vi "BusyLock.vi"(7 "BusyLock":refnum<vi>, 9 "Timeout(250)":i32=250, 10 "ExitEvent":refnum<user-event>, 11 "Counter":refnum<vi>) -> ()   [LabVIEW 2021, in "YActor.lvclass"]
uses:
  YActor.lvclass
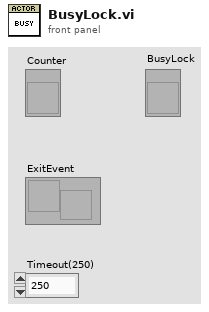
[diagram p1: front panel]
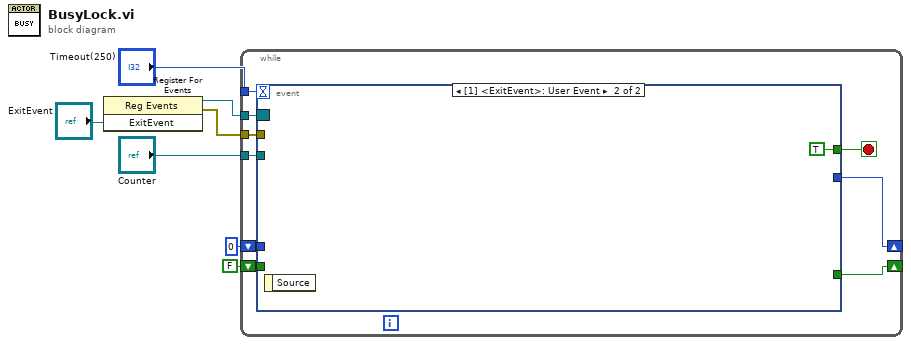
[diagram p0: block diagram]
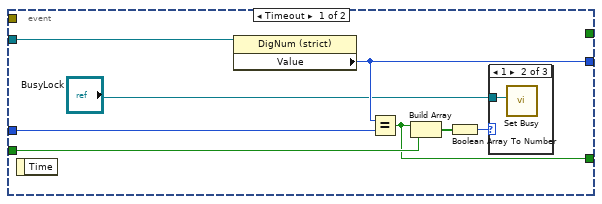
[diagram p2: hidden frame]
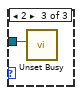
[diagram p4: hidden frame]
diagram:
  n1 = register-events("ExitEvent") -> (reference out=w3:refnum<event-registration>, error out=w1:errorcluster)  [unwired: 2 in]
  n2 = while {
    tunnel: w3 -> [w16]
    shift-right: [w13] -> _
    shift-left: 0 ("l_counter") -> [w14]
    shift-right: [w11] -> _
    shift-left: FALSE -> [w12]
    tunnel: "Timeout(250)" -> [w10]
    tunnel: "Counter" -> [w9]
    tunnel: w1 -> [w8]
    stop <- w15 stop-if-true
    n3 = event shown="[1] <ExitEvent>: User Event" {
      selector: w16 -> [_ _]
      dyn-events: _ -> [_ _]
      timeout: w10 -> [_ _]
      tunnel: [_ TRUE] -> w15
      tunnel: w14 -> [w24 _]
      tunnel: [w23 _] -> w13
      tunnel: w12 -> [w20 _]
      tunnel: [w19 _] -> w11
      tunnel: w9 -> [w18 _]
      tunnel: w8 -> [_ _]
      event Timeout {
        n4 = event-data() -> ()  [unwired: 1 in, 1 out]
        n5 = property class="DigNum (strict)"(reference=w18) -> ("Value"=w23:i32)  [unwired: 1 in, 2 out]
        n6 = Equal?(x=w23, y=w24) -> (x = y?=w19:bool)
        n7 = Build Array(w19, w20) -> (w22:bool[])
        n8 = Boolean Array To Number(Boolean array=w22) -> (number=w21:u32)
        n9 = case shown="1" w21 {
          tunnel: "BusyLock" -> [_ w25 w26]
          frame 0, Default {
          }
          frame 1 {
            n10 = call <vilib>:"Set Busy.vi"("VI reference (current VI)"=w25) -> ()  [unwired: 9 in, 2 out]
          }
          frame 2 {
            n11 = call <vilib>:"Unset Busy.vi"("VI reference (current VI)"=w26) -> ()  [unwired: 10 in, 1 out]
          }
        }
      }
      event User Event {
        n12 = event-data() -> ()  [unwired: 1 in, 1 out]
      }
    }
  }
